vi "ecg-mcsharry.vi"() -> ()   [LabVIEW 2025]
uses:
  <vilib>/numeric/Random Number (Range) DBL.vi
  <vilib>/Analysis/2dsp.llb/Inverse Complex FFT.vi
  <vilib>/Analysis/NI_AALPro.lvlib
panel:
  out "R-R time interval":waveform(dbl)(graph)
  out "wfm1+wfm2":waveform(dbl)(graph)
  in  "stop":bool
  in  "c1":dbl(slide)=0.010256410256410256 scale=0.0..1.0
  in  "f1":dbl(slide)=0.1076923076923077 scale=0.0..1.0
  in  "f2":dbl(slide)=0.2512820512820513 scale=0.0..1.0
  in  "c2":dbl(slide)=0.010256410256410256 scale=0.0..1.0
  in  "s2":dbl(slide)=0.06153846153846154 scale=0.0..1.0
  in  "s1":dbl(slide)=0.08717948717948718 scale=0.0..1.0
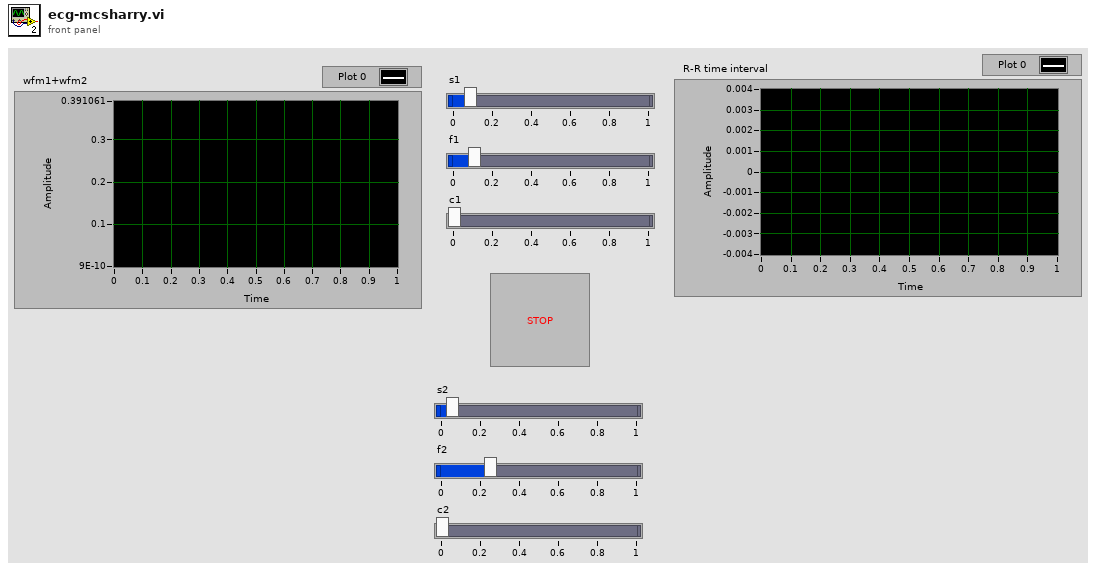
[diagram p1: front panel]
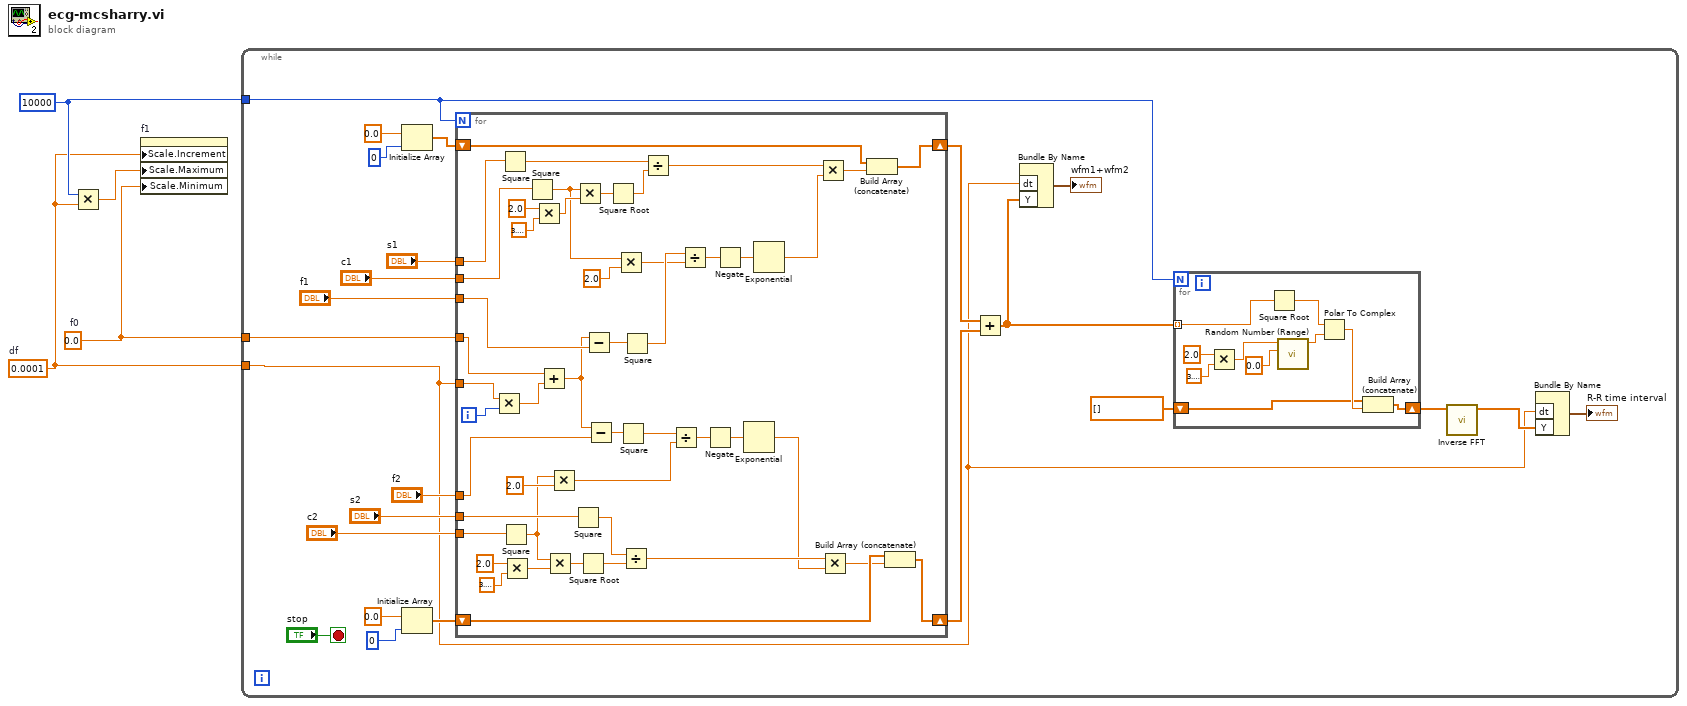
[diagram p0: block diagram]
diagram:
  w3 = 10000
  w1 = 0.0001  # df
  w4 = 0.0  # f0
  n1 = Multiply(x=w3, y=w1) -> (x*y=w2:dbl)
  n2 = property on="f1" class="Slide (strict)"("Scale.Increment"=w1, "Scale.Maximum"=w2, "Scale.Minimum"=w4) -> ()  [unwired: 2 in, 2 out]
  n3 = while {
    tunnel: w4 -> [w13]
    tunnel: w1 -> [w5]
    tunnel: w3 -> [w11]
    stop <- "stop" stop-if-true
    n4 = Initialize Array(0.0 ("element"), 0 ("dimension size")) -> (w28:dbl[])
    n5 = Initialize Array(0.0 ("element"), 0 ("dimension size")) -> (w14:dbl[])
    n6 = for {
      N: w11 -> [_]
      shift-right: [w65] -> w17
      shift-left: w28 -> [w64]
      shift-right: [w46] -> w16
      shift-left: w14 -> [w47]
      tunnel: "s1" -> [w85]
      tunnel: "c1" -> [w81]
      tunnel: "f1" -> [w73]
      tunnel: "s2" -> [w63]
      tunnel: "c2" -> [w53]
      tunnel: "f2" -> [w56]
      tunnel: w13 -> [w43]
      tunnel: w5 -> [w42]
      i -> [w77]
      n7 = Multiply(x=w42, y=w77) -> (x*y=w76:dbl)
      n8 = Square(x=w85) -> (x^2=w79:dbl)
      n9 = Square(x=w53) -> (x^2=w52:dbl)
      n10 = Multiply(x=2.0, y=3.141592653589793) -> (x*y=w59:dbl)
      n11 = Square(x=w81) -> (x^2=w71:dbl)
      n12 = Multiply(x=2.0, y=3.141592653589793) -> (x*y=w82:dbl)
      n13 = Add(x=w43, y=w76) -> (x+y=w40:dbl)
      n14 = Multiply(x=w52, y=w59) -> (x*y=w58:dbl)
      n15 = Multiply(x=w52, y=2.0) -> (x*y=w44:dbl)
      n16 = Square(x=w63) -> (x^2=w62:dbl)
      n17 = Multiply(x=w71, y=w82) -> (x*y=w80:dbl)
      n18 = Square Root(x=w58) -> (sqrt(x)=w57:dbl)
      n19 = Subtract(x=w40, y=w73) -> (x-y=w75:dbl)
      n20 = Subtract(x=w40, y=w56) -> (x-y=w55:dbl)
      n21 = Square Root(x=w80) -> (sqrt(x)=w78:dbl)
      n22 = Multiply(x=w71, y=2.0) -> (x*y=w69:dbl)
      n23 = Square(x=w55) -> (x^2=w45:dbl)
      n24 = Divide(x=w62, y=w57) -> (x/y=w49:dbl)
      n25 = Square(x=w75) -> (x^2=w72:dbl)
      n26 = Divide(x=w79, y=w78) -> (x/y=w74:dbl)
      n27 = Divide(x=w45, y=w44) -> (x/y=w50:dbl)
      n28 = Divide(x=w72, y=w69) -> (x/y=w67:dbl)
      n29 = Negate(x=w50) -> (-x=w51:dbl)
      n30 = Negate(x=w67) -> (-x=w68:dbl)
      n31 = Exponential(1:w51) -> (0:w48:dbl)
      n32 = Exponential(1:w68) -> (0:w66:dbl)
      n33 = Multiply(x=w74, y=w66) -> (x*y=w39:dbl)
      n34 = Multiply(x=w49, y=w48) -> (x*y=w41:dbl)
      n35 = Build Array (concatenate)(w64, w39) -> (w65:dbl[])
      n36 = Build Array (concatenate)(w47, w41) -> (w46:dbl[])
    }
    n37 = Add(x=w17, y=w16) -> (x+y=w9:dbl[])
    n38 = Bundle By Name("dt"=w5, "Y"=w9) -> (→"wfm1+wfm2":waveform(dbl))  [unwired: 1 in]
    n39 = for {
      N: w11 -> [_]
      tunnel: w9 -> [w29] mode=indexing
      shift-right: [w32] -> w10
      shift-left: cdb[] [] -> [w31]
      n40 = Multiply(x=2.0, y=3.141592653589793) -> (x*y=w36:dbl)
      n41 = Square Root(x=w29) -> (sqrt(x)=w30:dbl)
      n42 = call-poly <vilib>:"Random Number (Range).vi"("lower bound (0)"=0.0, "upper bound (100)"=w36) -> ("number"=w35:dbl)  [unwired: 9 in]
      n43 = Polar To Complex(1:w35, 2:w30) -> (0:w33:cdb)
      n44 = Build Array (concatenate)(w31, w33) -> (w32:cdb[])
    }
    n45 = call-poly <vilib>:"Inverse FFT.vi"("FFT {X}"=w10) -> ("X"=w6:cdb[])  [unwired: 9 in, 1 out]
    n46 = Bundle By Name("dt"=w5, "Y"=w6) -> (→"R-R time interval":waveform(cdb))  [unwired: 1 in]
  }
